vi "toml_parse_throwaway.vi"(11 "string in":string) -> (2 "comments":string, 3 "string out":string)   [LabVIEW 2017]
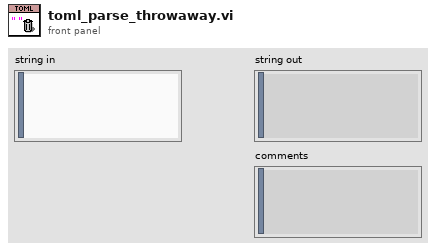
[diagram p1: front panel]
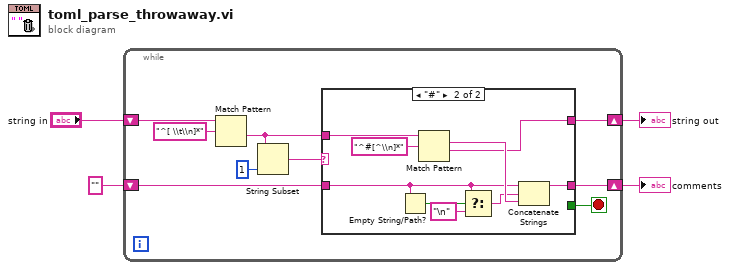
[diagram p0: block diagram]
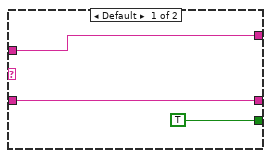
[diagram p2: hidden frame]
diagram:
  n1 = while {
    shift-right: [w7] -> w1
    shift-left: "" -> [w8]
    shift-right: [w5] -> w2
    shift-left: "string in" -> [w10]
    stop <- w6 stop-if-true
    n2 = Match Pattern(string=w10, regular expression="^[ \\t\\n]*") -> (after substring=w11:string)  [unwired: 1 in, 3 out]
    n3 = String Subset(string=w11, length (rest)=1 ("length (rest)")) -> (substring=w9:string)  [unwired: 1 in]
    n4 = case shown="\"#\"" w9 {
      tunnel: w11 -> [w14 w24]
      tunnel: w8 -> [w16 w18]
      tunnel: [w16 w23] -> w7
      tunnel: [TRUE _] -> w6
      tunnel: [w14 w21] -> w5
      frame Default {
      }
      frame "#" {
        n5 = Empty String/Path?(string/path=w18) -> (empty?=w20:bool)
        n6 = Match Pattern(string=w24, regular expression="^#[^\\n]*") -> (match substring=w22:string, after substring=w21:string)  [unwired: 1 in, 2 out]
        n7 = Select(t=w18, s=w20, f="\n") -> (s? t:f=w19:string)
        n8 = Concatenate Strings(w18, w19, w22) -> (w23:string)
      }
    }
  }
  "string out" <- w2
  "comments" <- w1
